vi "LV8_10c.vi"() -> ()   [LabVIEW 2014]
uses:
  <vilib>/imath/engines/lvmath2/RunTimeEngine/RangeToken/NIMS_Range.vi
  <instcachedir>/0/NIMS_Range_9BCE657718DF4976A877346C61F22738.lvgen/NIMS_Range_9BCE657718DF4976A877346C61F22738_000.vi
  <vilib>/imathl/engines/lvmath/Functions/Error Handling/Create Error.vi
  <vilib>/imath/engines/lvmath2/RunTimeEngine/BuiltInFunctions/round/NIMS_round(DBL-S).vi
  <vilib>/imath/engines/lvmath2/RunTimeEngine/BuiltInFunctions/fft/NIMS_fft(GV).vi
  <instcachedir>/0/NIMS_fft(GV)_4C6467FC22F84E4BA42517A07EF978B0.lvgen/NIMS_fft(GV)_4C6467FC22F84E4BA42517A07EF978B0_000.vi
  <vilib>/imath/engines/lvmath2/RunTimeEngine/BuiltInFunctions/abs/NIMS_abs(signed).vi
  <instcachedir>/0/NIMS_abs(signed)_C4FCB8E6058B49B797C7C8D53CA5F6EC.lvgen/NIMS_abs(signed)_C4FCB8E6058B49B797C7C8D53CA5F6EC_006.vi
  <vilib>/imath/engines/lvmath2/RunTimeEngine/ErrorHandling/NIMS_Error From Error Code.vi
  <vilib>/imath/engines/lvmath2/RunTimeSupport/NIMS_Error if Not Equal.vi
  <instcachedir>/0/NIMS_Error if Not Equal_8A0E9F659B9142D69417CC259581C4FD.lvgen/NIMS_Error if Not Equal_8A0E9F659B9142D69417CC259581C4FD_001.vi
  <vilib>/imath/engines/lvmath2/RunTimeEngine/IndexRead/NIMS V(V).vi
  <instcachedir>/0/NIMS V(V)_298D9CB7BFEB42B8BC8D9C3C28AE8C70.lvgen/NIMS V(V)_298D9CB7BFEB42B8BC8D9C3C28AE8C70_000.vi
  <vilib>/imath/engines/lvmath2/RunTimeEngine/ErrorHandling/NIMS_Create Error From Enums.vi
  <vilib>/imath/engines/lvmath2/RunTimeEngine/NodeEndStatement/NIMS_NodeEndStatement_Output.vi
  <instcachedir>/0/NIMS_NodeEndStatement_Output_53EC0D466D134D7ABD903AC30B43404B.lvgen/NIMS_NodeEndStatement_Output_53EC0D466D134D7ABD903AC30B43404B_005.vi
  <vilib>/imath/engines/lvmath2/RunTimeEngine/ErrorHandling/NIMS_Finalize Error.vi
panel:
  in  "Stop Button":bool
  in  "Fmax":dbl(slide) scale=5.0..10.0
  in  "Tmax":dbl(slide) scale=5.0..10.0
  out "Signal (time domain)":cluster{"T":dbl[], "X":dbl[]}(graph)
  out "Signal (frequency domain)":cluster{"F":dbl[], "FX":dbl[]}[](graph)
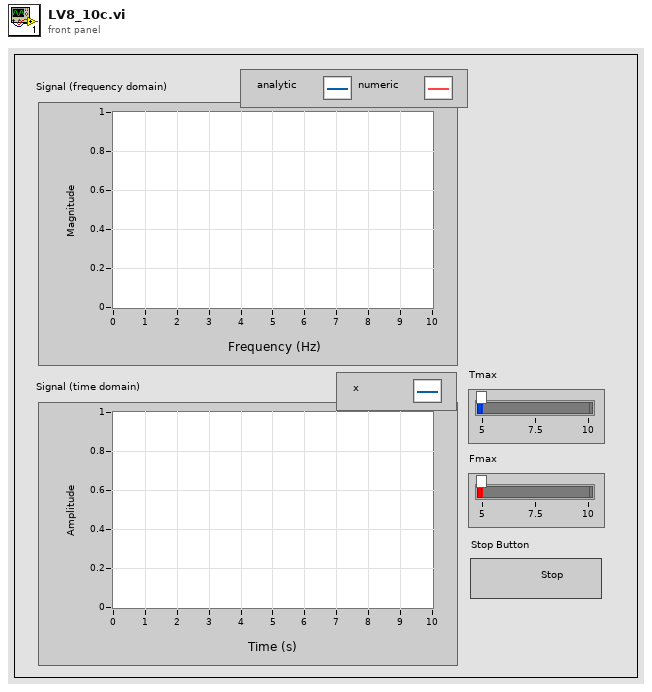
[diagram p1: front panel]
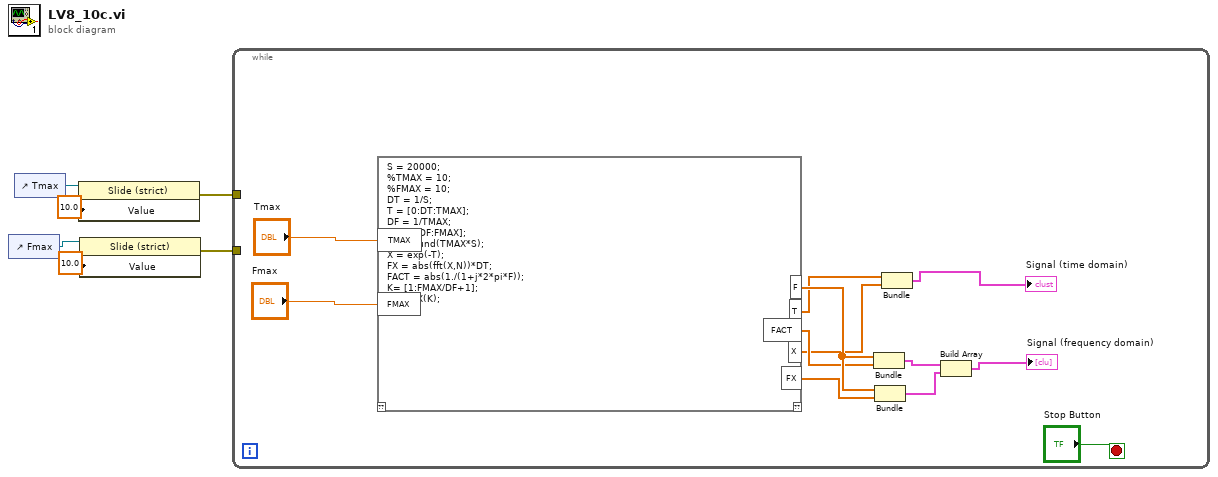
[diagram p0: block diagram]
diagram:
  n1 = control-ref of="Fmax"() -> (w2:refnum<vi>)
  n2 = control-ref of="Tmax"() -> (w6:refnum<vi>)
  n3 = property class="Slide (strict)"(reference=w6, "Value"=10.0) -> (error out=w5:errorcluster)  [unwired: 1 in, 1 out]
  n4 = property class="Slide (strict)"(reference=w2, "Value"=10.0) -> (error out=w1:errorcluster)  [unwired: 1 in, 1 out]
  n5 = while {
    tunnel: w5 -> [_]
    tunnel: w1 -> [_]
    stop <- "Stop Button" stop-if-true
    n6 = mathscript code="S = 20000;\n%TMAX = 10;\n%FMAX = 10;\nDT = 1/S;\nT = [0:DT:TMAX];\nDF = 1/TMAX;\nF = [0:DF:FMAX];\nN = round(TMAX*S);\nX = exp(-T);\nFX = abs(fft(X,N))*DT;\nFACT = abs(1./(1+j*2*pi*F));\nK= [1:FMAX/DF+1];\nFX = FX(K);"("TMAX"="Tmax", "FMAX"="Fmax") -> ("F"=w14:dbl[], "X"=w11:dbl[], "FX"=w15:dbl[], "T"=w12:dbl[], "FACT"=w13:dbl[])  [unwired: 1 in, 1 out]
    n7 = Bundle("F"=w14, "FACT"=w13) -> (w9:cluster{"F":dbl[], "FACT":dbl[]})  [unwired: 1 in]
    n8 = Bundle("F"=w14, "FX"=w15) -> (w8:cluster{"F":dbl[], "FX":dbl[]})  [unwired: 1 in]
    n9 = Bundle("T"=w12, "X"=w11) -> (→"Signal (time domain)":cluster{"T":dbl[], "X":dbl[]})  [unwired: 1 in]
    n10 = Build Array(w9, w8) -> (→"Signal (frequency domain)":cluster{"F":dbl[], "FX":dbl[]}[])
  }
